vi "test_Path (absolute).vi"(8 "error in (no error)":errorcluster, 11 "TestCase in":refnum<class "Test Read File.lvclass">) -> (0 "error out":errorcluster, 3 "TestCase out":refnum<class "Test Read File.lvclass">)   [LabVIEW 2019, in "Test Read File.lvclass"]
uses:
  Test Read File.lvclass
  C:/Program Files/National Instruments/LabVIEW 2024/vi.lib/Astemes/LUnit/Test Case.lvclass
  Test Read File.lvclass/Test Read File.ctl
  <vilib>/Astemes/LUnit/Test Case.lvclass/Test Case.ctl
  6e6e6e9d-8f5f-49ca-813c-84131d19af41.vi
  <vilib>/Astemes/LUnit/Core/LUnit Test Case/Private/Append Pass Result.vi
  <vilib>/Astemes/LUnit/Core/LUnit Test Case/Private/Append Fail Result.vi
  6e6e6e9d-8f5f-49ca-813c-84131d19af41.vi/9c5d11cd-9439-4240-a1ee-d9baace9c924.vi
  <vilib>/Astemes/LUnit/Core/LUnit Test Case/Private/Run In UI.vi
  <vilib>/Utility/error.llb/Clear Errors.vi
  Read/Read Section - Path.vi
  TSC File IO.lvlib
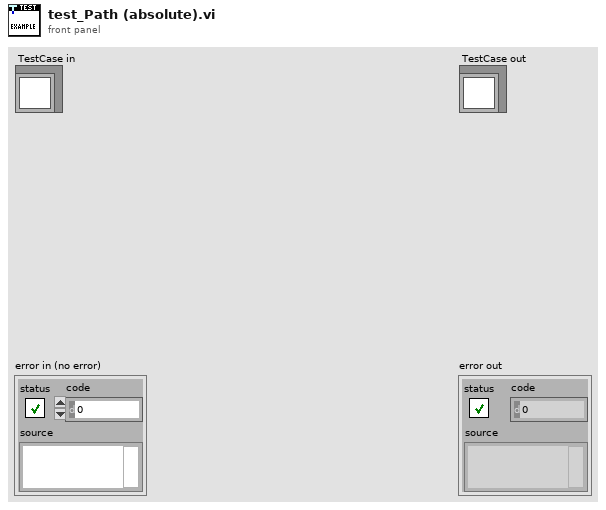
[diagram p1: front panel]
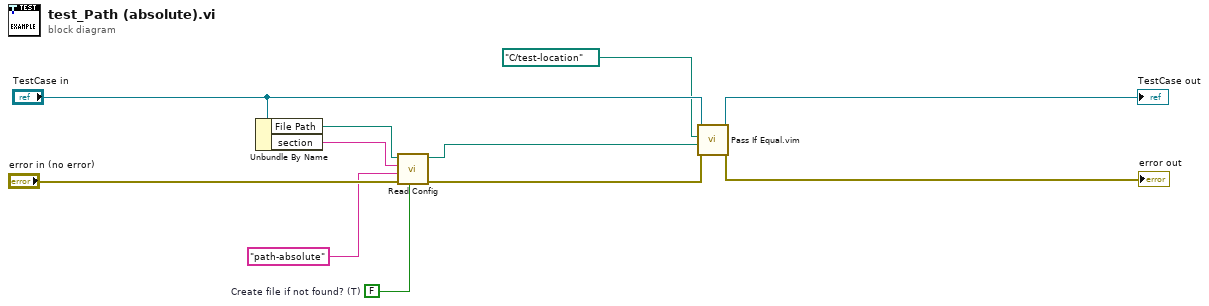
[diagram p0: block diagram]
diagram:
  w6 = FALSE  # Create file if not found? (T)
  n1 = Unbundle By Name("TestCase in") -> ("File Path"=w1:path, "section"=w2:string)
  n2 = call-poly "Read Config.vi"("Create file if not found? (T)"=w6, "error in (no error)"="error in (no error)", "key"="path-absolute", "section"=w2, "Path"=w1) -> ("error out"=w5:errorcluster, "value"=w4:path)  [unwired: 5 in]
  n3 = call "Pass If Equal.vim"("error in (no error)"=w5, "Actual"=w4, "Expected"=path "C:/test-location", "LUnit Test Case In"="TestCase in") -> ("error out"=→"error out":errorcluster, "LUnit Test Case Out"=→"TestCase out":refnum<class "Test Read File.lvclass">)  [unwired: 6 in]
